vi "Initialize Sink.vi"(11 "Buffered Log Sink in":refnum<class "Buffered String Log Sink.lvclass">) -> (0 "error out":errorcluster, 3 "Buffered Log Sink out":refnum<class "Buffered String Log Sink.lvclass">)   [LabVIEW 2020, in "MVA Framework.lvlib" / "Buffered String Log Sink.lvclass"]
uses:
  Buffered String Log Sink.lvclass
  Buffered String Log Sink.lvclass/Buffered String Log Sink.ctl
  String Log Sink/String Log Sink.lvclass
  Timeout Watchdog.vi
  Composed Log/Log Sink/Log Sink.lvclass
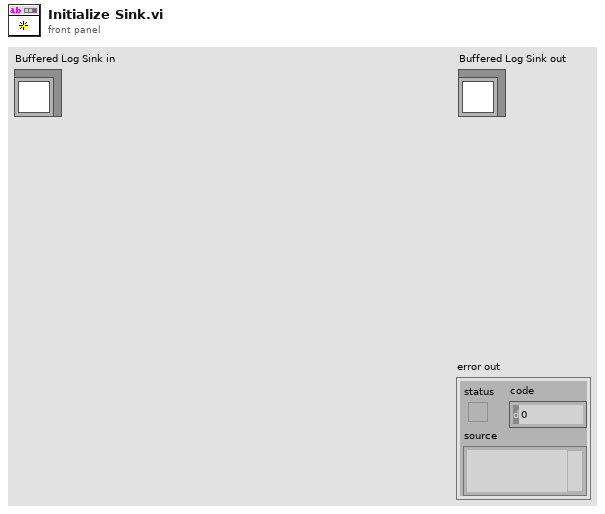
[diagram p1: front panel]
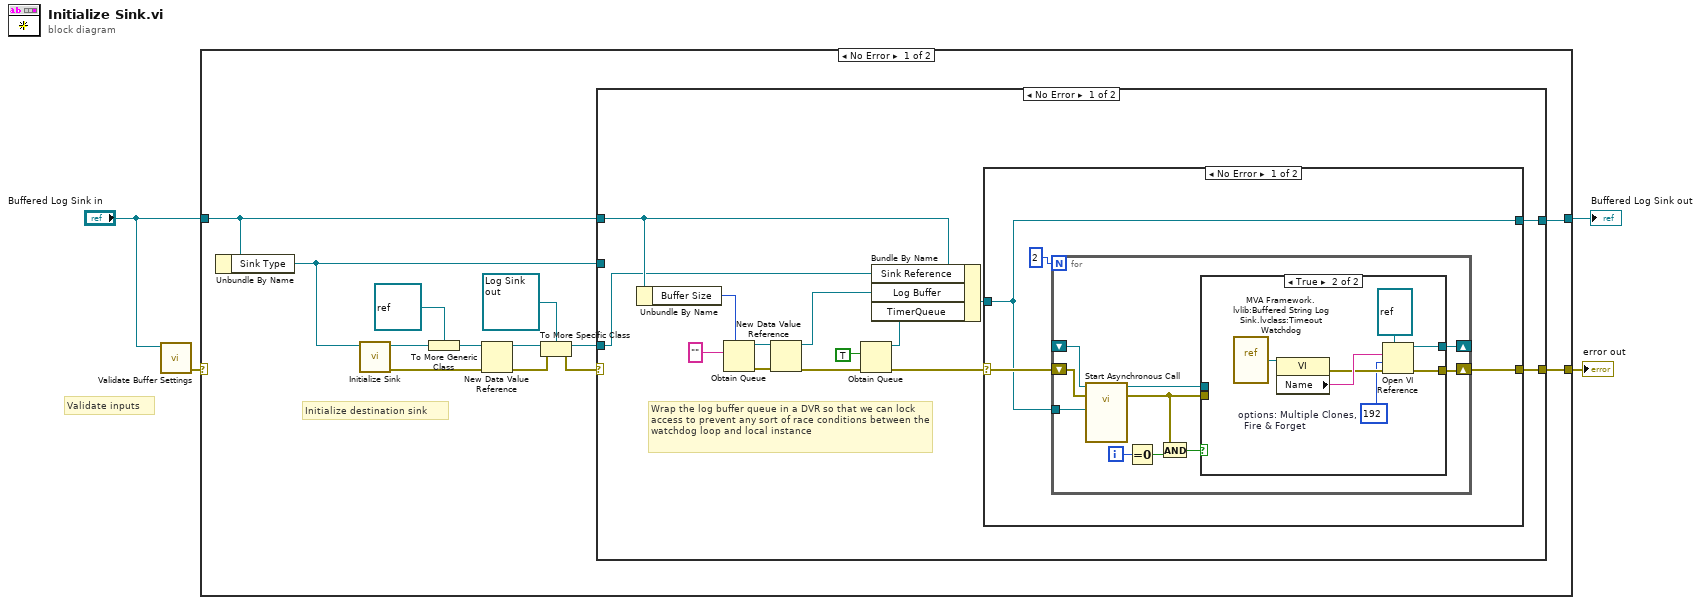
[diagram p0: block diagram]
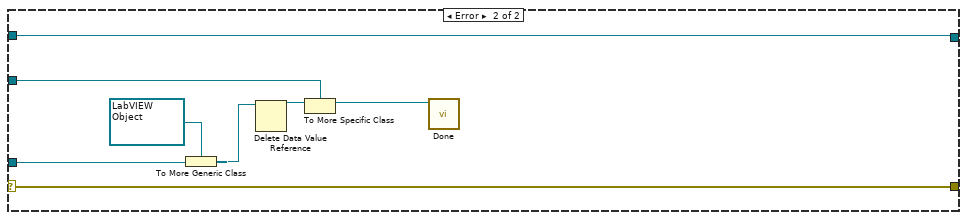
[diagram p4: hidden frame]
diagram:
  # "Validate inputs"
  n1 = call "Validate Buffer Settings.vi"("Buffered Log Sink in"="Buffered Log Sink in") -> ("error out"=w1:errorcluster)  [unwired: 10 in]
  n2 = case shown="No Error" w1 {
    selector: w1 -> [_ w65]
    tunnel: [w17 w66] -> w4
    tunnel: [w16 w65] -> w3
    tunnel: "Buffered Log Sink in" -> [w14 w66]
    frame No Error {
      # "Initialize destination sink"
      n3 = Unbundle By Name(w14) -> ("Sink Type"=w5:refnum<class "Log Sink.lvclass">)
      n4 = call-dynamic "Initialize Sink.vi"("Log Sink in"=w5) -> ("error out"=w13:errorcluster, "Log Sink out"=w9:refnum<class "Log Sink.lvclass">)  [unwired: 9 in]
      n5 = To More Generic Class(target class=refnum<class> refnum ("LabVIEW Object"), reference=w9) -> (generic class reference=w7:refnum<class>)
      n6 = New Data Value Reference(data value=w7, error in=w13) -> (data value reference=w6:refnum<data-value>, error out=w12:errorcluster)
      n7 = To More Specific Class(target class=refnum<data-value> refnum ("data value reference"), reference=w6, error in=w12) -> (specific class reference=w10:refnum<data-value>, error out=w11:errorcluster)
      n8 = case shown="No Error" w11 {
        selector: w11 -> [_ w63]
        tunnel: [w23 w64] -> w17
        tunnel: [w22 w63] -> w16
        tunnel: w14 -> [w21 w64]
        tunnel: w10 -> [w20 w61]
        tunnel: w5 -> [_ w62]
        frame No Error {
          # "Wrap the log buffer queue in a DVR so that we can lock access to prevent any sort of race conditions between the watchdog loop and local instance"
          n9 = Unbundle By Name(w21) -> ("Buffer Size"=w27:i32)
          n10 = Obtain Queue(max queue size (-1, unlimited)=w27, element data type="") -> (queue out=w28:refnum<queue>, error out=w26:errorcluster)  [unwired: 3 in, 1 out]
          n11 = New Data Value Reference(data value=w28, error in=w26) -> (data value reference=w18:refnum<data-value>, error out=w25:errorcluster)
          n12 = Obtain Queue(element data type=TRUE, error in (no error)=w25) -> (queue out=w29:refnum<queue>, error out=w24:errorcluster)  [unwired: 3 in, 1 out]
          n13 = Bundle By Name(cluster=w21, "Sink Reference"=w20, "Log Buffer"=w18, "TimerQueue"=w29) -> (w30:refnum<class "Buffered String Log Sink.lvclass">)
          n14 = case shown="No Error" w24 {
            selector: w24 -> [w34 w55]
            tunnel: w30 -> [w33 w56]
            tunnel: [w33 w56] -> w23
            tunnel: [w32 w55] -> w22
            frame No Error {
              n15 = for {
                N: 2 -> [_]
                shift-right: [w41] -> _
                shift-left: _ -> [w45]
                tunnel: w33 -> [w37]
                shift-right: [w39] -> w32
                shift-left: w34 -> [w36]
                i -> [w44]
                n16 = call-by-ref "Start Asynchronous Call"(reference=w45, error in=w36, "Buffered Log Sink in"=w37) -> (reference out=w42:refnum<vi>, error out=w38:errorcluster)  [unwired: 11 in]
                n17 = Equal To 0?(x=w44) -> (x = 0?=w43:bool)
                n18 = And(x=w38, y=w43) -> (x .and. y?=w40:bool)
                n19 = case shown="True" w40 {
                  tunnel: w42 -> [w47 _]
                  tunnel: [w46 w50] -> w39
                  tunnel: [w47 w49] -> w41
                  tunnel: w38 -> [w46 _]
                  frame False {
                  }
                  frame True {
                    w48 = 192  # options: Multiple Clones,   Fire & Forget
                    n20 = vi-ref "MVA Framework.lvlib:Buffered String Log Sink.lvclass:Timeout Watchdog.vi"() -> (w52:refnum<vi>)
                    n21 = property class="VI"(reference=w52) -> (error out=w53:errorcluster, "Name"=w54:string)  [unwired: 1 in, 1 out]
                    n22 = Open VI Reference(type specifier VI Refnum (for type only)=refnum<vi> refnum, vi path=w54, options=w48, error in (no error)=w53) -> (vi reference=w49:refnum<vi>, error out=w50:errorcluster)  [unwired: 2 in]
                  }
                }
              }
            }
            frame Error {
            }
          }
        }
        frame Error {
          n23 = To More Generic Class(target class=refnum<data-value> refnum ("data value reference"), reference=w61) -> (generic class reference=w59:refnum<data-value>)
          n24 = Delete Data Value Reference(data value reference=w59) -> (data value=w58:refnum<class>)  [unwired: 1 in, 1 out]
          n25 = To More Specific Class(target class=w62, reference=w58) -> (specific class reference=w57:refnum<class "Log Sink.lvclass">)  [unwired: 1 in, 1 out]
          n26 = call-dynamic "Done.vi"("Log Sink in"=w57) -> ()  [unwired: 10 in, 1 out]
        }
      }
    }
    frame Error {
      # "Invalid buffer settings"
    }
  }
  "error out" <- w3
  "Buffered Log Sink out" <- w4
